vi "Spike LED Test.vi"(9 "Climb":bool, 10 "Spun up":bool, 11 "Spike":T1={"DevStatus"={"status"=FALSE, "code"=0, "source"=""}, "Relay Channel"=enum."Invalid", "Digital Module"=enum."Digital Module 1", "Relay Direction"=enum."Both directions"}) -> ()   [LabVIEW 2012]
uses:
  <vilib>/Rock Robotics/WPI/Relay/WPI_RelayDevRef.ctl
  <vilib>/Rock Robotics/SystemInterfaces/DIO/FPGA_DIORelayChannel.ctl
  <vilib>/Rock Robotics/SystemInterfaces/Typedef/FPGA_TypedefDigitalModule.ctl
  <vilib>/Rock Robotics/WPI/Relay/WPI_RelayDirection.ctl
  <vilib>/Rock Robotics/WPI/Relay/WPI_RelayValue.ctl
  Globals/Useful Values.vi
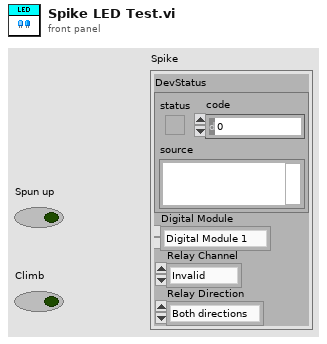
[diagram p1: front panel]
types:
  T1 = typedef "WPI_RelayDevRef.ctl" = cluster{"DevStatus":errorcluster, "Relay Channel":T2, "Digital Module":T3, "Relay Direction":T4}
  T2 = typedef "FPGA_DIORelayChannel.ctl" = enum8{"Relay 1", "Relay 2", "Relay 3", "Relay 4", "Relay 5", "Relay 6", "Relay 7", "Relay 8", "Invalid"}
  T3 = typedef "FPGA_TypedefDigitalModule.ctl" = enum16{"Digital Module 1", "Digital Module 2"}
  T4 = typedef "WPI_RelayDirection.ctl" = enum16{"Both directions", "Forward only", "Reverse only"}
  T5 = typedef "WPI_RelayValue.ctl" = enum16{"Off", "On", "Forward", "Reverse"}
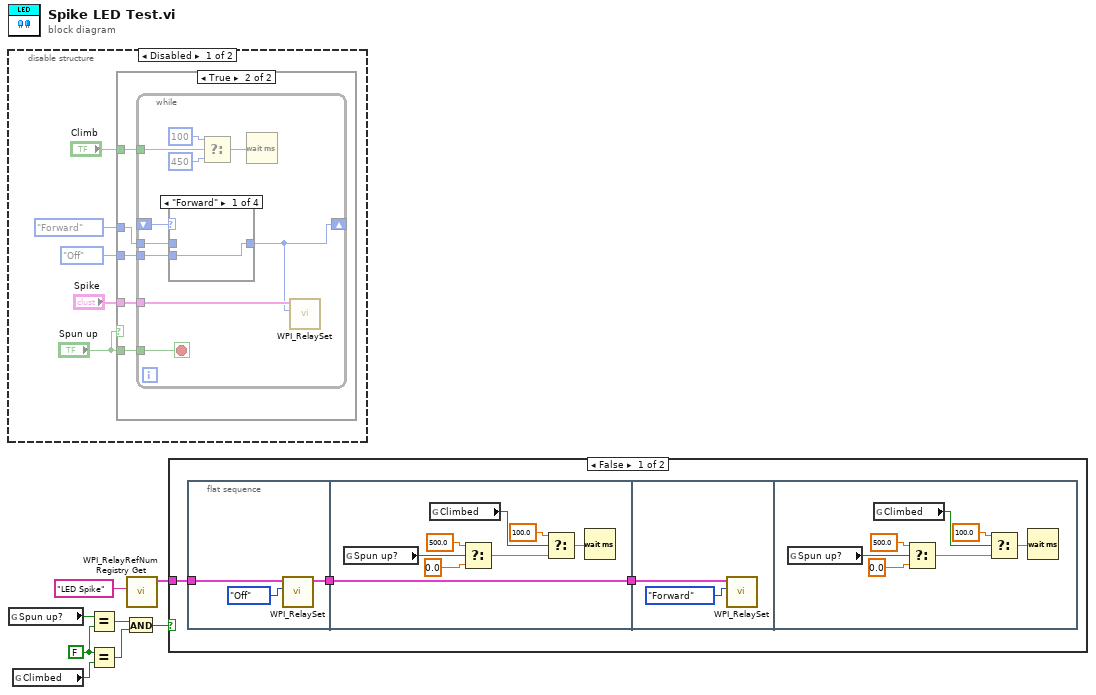
[diagram p0: block diagram]
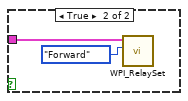
[diagram p2: hidden frame]
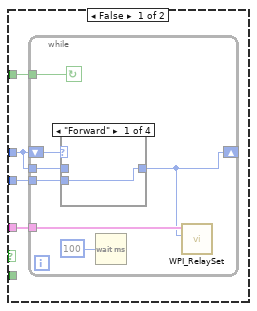
[diagram p3: hidden frame]
diagram:
  w6 = FALSE
  n1 = disable-structure shown="Disabled" {
    frame Disabled {
      n2 = case shown="True" "Spun up" {
        tunnel: "Spike" -> [w16 w30]
        tunnel: WPI_RelayValue."Off" ("RelayValue") -> [w15 w33]
        tunnel: WPI_RelayValue."Forward" ("RelayValue") -> [w14 w32]
        tunnel: "Spun up" -> [_ w31]
        tunnel: "Climb" -> [w17 w29]
        frame False {
          n3 = while {
            tunnel: w17 -> [w24]
            tunnel: w16 -> [w22]
            shift-right: [w18] -> _
            shift-left: w14 -> [w21]
            tunnel: w15 -> [w20]
            tunnel: w14 -> [w19]
            stop <- w24 continue-if-true
            n4 = case shown="\"Forward\"" w21 {
              tunnel: w20 -> [w25 _ w27 _]
              tunnel: w19 -> [_ w26 _ w28]
              tunnel: [w25 w26 w27 w28] -> w18
              frame "Forward" {
              }
              frame "Reverse" {
              }
              frame "On" {
              }
              frame "Off" {
              }
            }
            n5 = Wait (ms)(milliseconds to wait=u32 100 ("t")) -> ()  [unwired: 1 out]
            n6 = call <vilib>:"WPI_RelaySet.vi"("RelayValue"=w18, "RelayDevRef"=w22) -> ()  [unwired: 8 in, 2 out]
          }
        }
        frame True {
          n7 = while {
            tunnel: w31 -> [w43]
            tunnel: w32 -> [w41]
            tunnel: w33 -> [w42]
            shift-right: [w38] -> _
            shift-left: _ -> [w40]
            tunnel: w30 -> [w39]
            tunnel: w29 -> [w37]
            stop <- w43 stop-if-true
            n8 = case shown="\"Forward\"" w40 {
              tunnel: w42 -> [w44 _ w46 _]
              tunnel: w41 -> [_ w45 _ w47]
              tunnel: [w44 w45 w46 w47] -> w38
              frame "Forward" {
              }
              frame "Reverse" {
              }
              frame "On" {
              }
              frame "Off" {
              }
            }
            n9 = Select(t=u32 100, s=w37, f=u32 450 ("milliseconds to wait")) -> (s? t:f=w34:u32)
            n10 = Wait (ms)(milliseconds to wait=w34) -> ()  [unwired: 1 out]
            n11 = call <vilib>:"WPI_RelaySet.vi"("RelayValue"=w38, "RelayDevRef"=w39) -> ()  [unwired: 8 in, 2 out]
          }
        }
      }
    }
    frame Enabled {
    }
  }
  n12 = global read "Useful Values.vi" "Spun up?"() -> (w7:bool)
  n13 = global read "Useful Values.vi" "Climbed"() -> (w5:bool)
  n14 = Equal?(x=w7, y=w6) -> (x = y?=w4:bool)
  n15 = Equal?(x=w6, y=w5) -> (x = y?=w3:bool)
  n16 = And(x=w4, y=w3) -> (x .and. y?=w1:bool)
  n17 = call <vilib>:"WPI_RelayRefNum Registry Get.vi"("refnum name"="LED Spike") -> ("RelayDevRef"=w2:T1)  [unwired: 9 in, 1 out]
  n18 = case shown="False" w1 {
    tunnel: w2 -> [w48 w72]
    frame False {
      n19 = flat-sequence {
        tunnel: w48 -> [w52]
        tunnel: [w51] -> w50
        tunnel: w50 -> [w56]
        tunnel: [w56] -> w49
        tunnel: w49 -> [w62]
        frame #0 {
          n20 = call <vilib>:"WPI_RelaySet.vi"("RelayValue"=WPI_RelayValue."Off", "RelayDevRef"=w52) -> ("RelayDevRef"=w51:T1)  [unwired: 8 in, 1 out]
        }
        frame #1 {
          n21 = global read "Useful Values.vi" "Spun up?"() -> (w54:bool)
          n22 = global read "Useful Values.vi" "Climbed"() -> (w59:bool)
          n23 = Select(t=500.0, s=w54, f=0.0) -> (s? t:f=w60:dbl)
          n24 = Select(t=100.0, s=w59, f=w60) -> (s? t:f=w61:dbl)
          n25 = Wait (ms)(milliseconds to wait=w61) -> ()  [unwired: 1 out]
        }
        frame #2 {
          n26 = call <vilib>:"WPI_RelaySet.vi"("RelayValue"=WPI_RelayValue."Forward", "RelayDevRef"=w62) -> ()  [unwired: 8 in, 2 out]
        }
        frame #3 {
          n27 = global read "Useful Values.vi" "Spun up?"() -> (w70:bool)
          n28 = global read "Useful Values.vi" "Climbed"() -> (w66:bool)
          n29 = Select(t=500.0, s=w70, f=0.0) -> (s? t:f=w65:dbl)
          n30 = Select(t=100.0, s=w66, f=w65) -> (s? t:f=w64:dbl)
          n31 = Wait (ms)(milliseconds to wait=w64) -> ()  [unwired: 1 out]
        }
      }
    }
    frame True {
      n32 = call <vilib>:"WPI_RelaySet.vi"("RelayValue"=WPI_RelayValue."Forward", "RelayDevRef"=w72) -> ()  [unwired: 8 in, 2 out]
    }
  }
